vi "Error Query.vi"(8 "error in (no error)":errorcluster, 11 "VISA resource name":refnum<visa-resource-name>) -> (0 "error out":errorcluster, 3 "VISA resource name out":refnum<visa-resource-name>)   [LabVIEW 2012]
doc: "Queries the instrument for any errors in the instrument's error queue. It will continue to read errors until all errors have been read from the instrument. Any errors will be returned in the <B>error out</B> control.\n\n<B>Note:</B>\nThis VI is called automatically by most driver VIs so it is not usually necessary to call this in an application."
panel:
  # "EDIT: Note: The Error Query VI is included as a subVI in all driver VIs except low-level API VIs. If the instrument does not support error query, then remove the VI and remove subVI calls in each instrument driver VI that calls it."
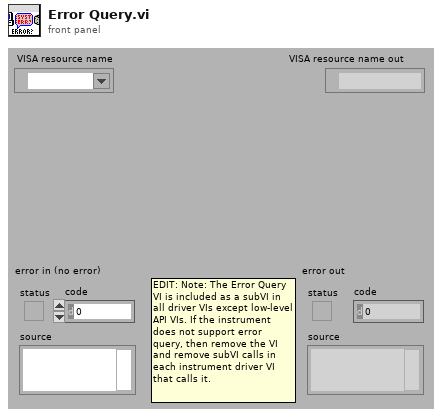
[diagram p1: front panel]
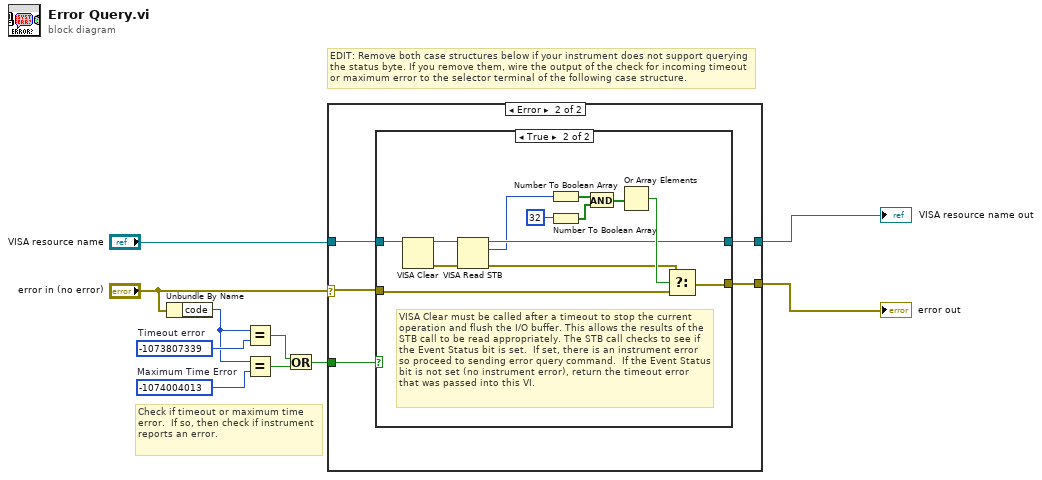
[diagram p0: block diagram]
diagram:
  w7 = -1074004013  # Maximum Time Error
  w9 = -1073807339  # Timeout error
  # "Check if timeout or maximum time error.  If so, then check if instrument reports an error."
  # "EDIT: Remove both case structures below if your instrument does not support querying the status byte. If you remove them, wire the output of the check for incoming timeout or maximum error to the selector terminal of the following case structure."
  n1 = Unbundle By Name("error in (no error)") -> ("code"=w8:i32)
  n2 = Equal?(x=w8, y=w9) -> (x = y?=w5:bool)
  n3 = Equal?(x=w8, y=w7) -> (x = y?=w6:bool)
  n4 = Or(x=w5, y=w6) -> (x .or. y?=w4:bool)
  n5 = case shown="Error" "error in (no error)" {
    selector: "error in (no error)" -> [w11 w15]
    tunnel: "VISA resource name" -> [w12 w17]
    tunnel: [w12 w16] -> w2
    tunnel: [w11 w14] -> w1
    tunnel: w4 -> [_ w13]
    frame No Error {
    }
    frame Error {
      n6 = case shown="True" w13 {
        tunnel: w17 -> [w19 w25]
        tunnel: [w19 w22] -> w16
        tunnel: w15 -> [w18 w28]
        tunnel: [w18 w27] -> w14
        frame False {
          # "Error code not a timeout, so best to pass on to user."
        }
        frame True {
          # "VISA Clear must be called after a timeout to stop the current operation and flush the I/O buffer. This allows the results of the  STB call to be read appropriately. The STB call checks to see if the Event Status bit is set.  If set, there is an instrument error so proceed to sending error query command.  If the Event Status bit is not set (no instrument error), return the timeout error that was passed into this VI."
          n7 = VISA Clear(VISA resource name=w25) -> (VISA resource name out=w24:refnum<visa-resource-name>, error out=w23:errorcluster)  [unwired: 1 in]
          n8 = VISA Read STB(8:w23, 11:w24) -> (0:w21:errorcluster, 2:w20:u16, 3:w22:refnum<visa-resource-name>)
          n9 = Number To Boolean Array(number=w20) -> (Boolean array=w29:bool[])
          n10 = Number To Boolean Array(number=32) -> (Boolean array=w31:bool[])
          n11 = And(x=w29, y=w31) -> (x .and. y?=w30:bool[])
          n12 = Or Array Elements(Boolean array=w30) -> (logical OR=w26:bool)
          n13 = Select(t=w21, s=w26, f=w28) -> (s? t:f=w27:errorcluster)
        }
      }
    }
  }
  "VISA resource name out" <- w2
  "error out" <- w1
